vi "Save VI.vi"(8 "error in (no error)":errorcluster, 11 "VI in":refnum<class "VI.lvclass">) -> (0 "error out":errorcluster, 3 "VI out":refnum<class "VI.lvclass">)   [LabVIEW 2015, in "VI.lvclass"]
uses:
  VI.lvclass
  VI.lvclass/VI.ctl
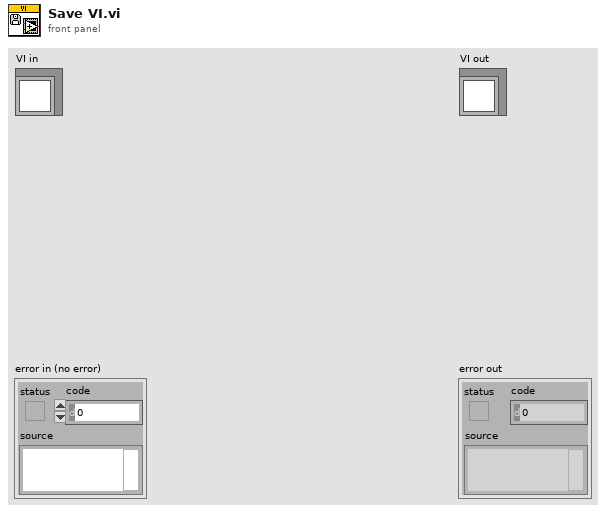
[diagram p1: front panel]
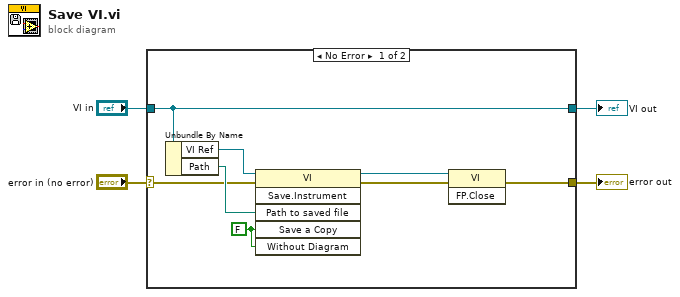
[diagram p0: block diagram]
diagram:
  n1 = case shown="No Error" "error in (no error)" {
    selector: "error in (no error)" -> [w8 w14]
    tunnel: [w5 w14] -> w3
    tunnel: [w12 w13] -> w1
    tunnel: "VI in" -> [w12 w13]
    frame No Error {
      w9 = FALSE ("Save a Copy")
      n2 = Unbundle By Name(w12) -> ("VI Ref"=w11:refnum<vi>, "Path"=w10:path)
      n3 = invoke class="VI" method="Save.Instrument"(reference=w11, error in=w8, "Path to saved file"=w10, "Save a Copy"=w9, "Without Diagram"=w9) -> (reference out=w7:refnum<vi>, error out=w6:errorcluster)  [unwired: 1 in, 4 out]
      n4 = invoke class="VI" method="FP.Close"(reference=w7, error in=w6) -> (error out=w5:errorcluster)  [unwired: 1 in, 2 out]
    }
    frame Error {
    }
  }
  "error out" <- w3
  "VI out" <- w1
